vi "convolve.vi"(0 "X":dbl[](array[numeric]) format="%.2f", 1 "Calc":u16(ring) items=["One way", "RT Single Rings", "R/T Full Aperture"], 2 "Y":dbl[](array[numeric]) format="%.2f", 3 "delay pts":i32) -> (5 "X*Y":dbl[](array[numeric]) format="%.2f")   [LabVIEW 2022 SP3]
uses:
  <vilib>/Analysis/2dsp.llb/Real FFT.vi
  <vilib>/Analysis/2dsp.llb/Inverse Complex FFT.vi
  <vilib>/Analysis/2dsp.llb/1D Convolution (DBL).vi
  <vilib>/Analysis/NI_AALPro.lvlib
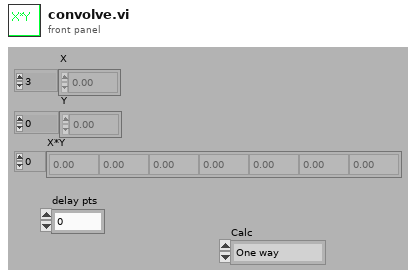
[diagram p1: front panel]
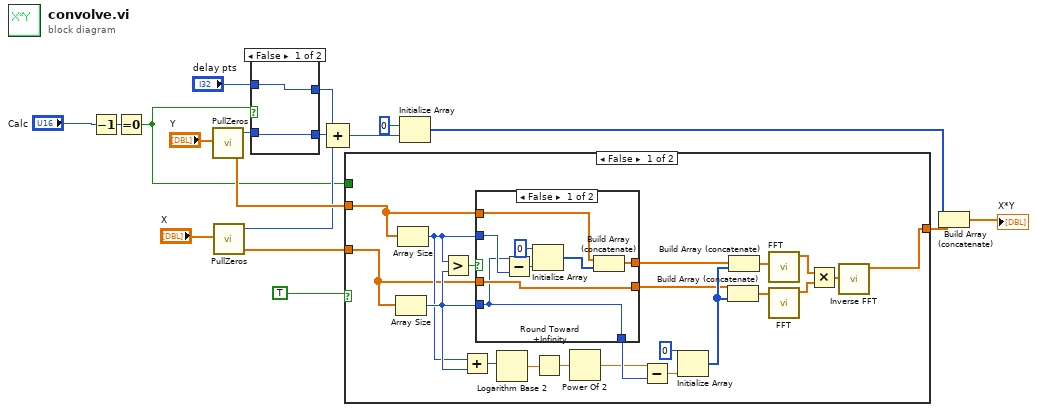
[diagram p0: block diagram]
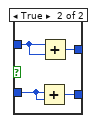
[diagram p2: hidden frame]
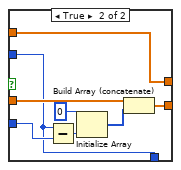
[diagram p3: hidden frame]
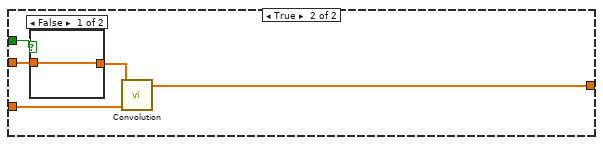
[diagram p4: hidden frame]
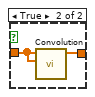
[diagram p5: hidden frame]
diagram:
  n1 = Decrement(x="Calc") -> (x-1=w4:u16)
  n2 = Equal To 0?(x=w4) -> (x = 0?=w3:bool)
  n3 = call "PullZeros.vi"("input"="Y") -> ("output"=w16:dbl[], "pre-zeros"=w10:i32)  [unwired: 3 out]
  n4 = call "PullZeros.vi"("input"="X") -> ("output"=w15:dbl[], "pre-zeros"=w14:i32)  [unwired: 3 out]
  n5 = case shown="False" w3 {
    tunnel: [w20 w21] -> w7
    tunnel: w10 -> [w20 w23]
    tunnel: [w19 w24] -> w8
    tunnel: "delay pts" -> [w19 w22]
    frame False {
    }
    frame True {
      n6 = Add(x=w23, y=w23) -> (x+y=w21:i32)
      n7 = Add(x=w22, y=w22) -> (x+y=w24:i32)
    }
  }
  n8 = Compound Arithmetic op=ADD(w8, w7, w14) -> (w17:i32)
  n9 = case shown="False" TRUE {
    tunnel: w16 -> [w27 w64]
    tunnel: w15 -> [w26 w62]
    tunnel: [w25 w66] -> w12
    tunnel: w3 -> [_ w65]
    frame False {
      n10 = Array Size(array=w26) -> (size(s)=w30:i32)
      n11 = Array Size(array=w27) -> (size(s)=w29:i32)
      n12 = Greater?(x=w29, y=w30) -> (0:w28:bool)
      n13 = Add(x=w29, y=w30) -> (x+y=w31:i32)
      n14 = case shown="False" w28 {
        tunnel: w29 -> [w49 w54]
        tunnel: w30 -> [w46 w61]
        tunnel: w26 -> [w47 w58]
        tunnel: [w47 w56] -> w36
        tunnel: w27 -> [w50 w55]
        tunnel: [w48 w55] -> w37
        tunnel: [w46 w54] -> w40
        frame False {
          n15 = Subtract(x=w46, y=w49) -> (x-y=w52:i32)
          n16 = Initialize Array(0, w52) -> (w51:i32[])
          n17 = Build Array (concatenate)(w50, w51) -> (w48:dbl[])
        }
        frame True {
          n18 = Subtract(x=w54, y=w61) -> (x-y=w59:i32)
          n19 = Initialize Array(0, w59) -> (w57:i32[])
          n20 = Build Array (concatenate)(w58, w57) -> (w56:dbl[])
        }
      }
      n21 = Logarithm Base 2(1:w31) -> (0:w32:dbl)
      n22 = Round Toward +Infinity(x=w32) -> (ceil(x): smallest int >= x=w33:dbl)
      n23 = Power Of 2(x=w33) -> (2^x=w39:dbl)
      n24 = Subtract(x=w39, y=w40) -> (x-y=w35:dbl)
      n25 = Initialize Array(0, w35) -> (w38:i32[])
      n26 = Build Array (concatenate)(w36, w38) -> (w45:dbl[])
      n27 = Build Array (concatenate)(w37, w38) -> (w44:dbl[])
      n28 = call-poly <vilib>:"FFT.vi"("X"=w44) -> ("FFT {X}"=w41:cdb[])  [unwired: 2 in, 8 out]
      n29 = call-poly <vilib>:"FFT.vi"("X"=w45) -> ("FFT {X}"=w42:cdb[])  [unwired: 2 in, 8 out]
      n30 = Multiply(x=w41, y=w42) -> (x*y=w43:cdb[])
      n31 = call-poly <vilib>:"Inverse FFT.vi"("FFT {X}"=w43) -> ("X"=w25:cdb[])  [unwired: 1 in, 9 out]
    }
    frame True {
      n32 = case shown="False" w65 {
        tunnel: [w67 w69] -> w63
        tunnel: w64 -> [w67 w68]
        frame False {
        }
        frame True {
          n33 = call-poly <vilib>:"Convolution.vi"("Y"=w68, "X"=w68) -> ("X * Y"=w69:dbl[])  [unwired: 1 in, 8 out]
        }
      }
      n34 = call-poly <vilib>:"Convolution.vi"("Y"=w62, "X"=w63) -> ("X * Y"=w66:dbl[])  [unwired: 1 in, 8 out]
    }
  }
  n35 = Initialize Array(0, w17) -> (w13:i32[])
  n36 = Build Array (concatenate)(w13, w12) -> (→"X*Y":cdb[])
